vi "After Launch Init.vi"(8 "error in (no error)":errorcluster, 11 "CS++BaseActor in":refnum<class "CS++BaseActor.lvclass">) -> (0 "error out":errorcluster, 3 "CS++BaseActor out":refnum<class "CS++BaseActor.lvclass">)   [LabVIEW 2015, in "CS++BaseActor.lvlib" / "CS++BaseActor.lvclass"]
doc: "Use <b>After Launch init.vi</b> method only for sanity checks that are supposed to prevent the actor from launching if they fail. Use <B>this</B> method instead to initialize unique resources that must be released during the <b>Stop Core.vi</b> method. A corresponding high priority message will become dispatched before the <B>Actor Framework.lvlib:Actor.lvclass.Actor Core.vi</b> is called.\n\n<b>Derived classed should call the parent methode first</b> and their own initialization code after.\n\nRefer also to the ongoing discussion at https://decibel.ni.com/content/message/57394#57394."
uses:
  CS++BaseActor.lvclass
  <vilib>/ActorFramework/Actor/Actor.lvclass/Actor.ctl
  <vilib>/ActorFramework/Message Enqueuer/Message Enqueuer.lvclass/Message Enqueuer.ctl
  CS++BaseActor.lvclass/CS++BaseActor.ctl
  Libraries/Base/FGV Action.ctl
  CS++BaseActor Messages/Polling Start Stop Msg/Polling Start Stop Msg.lvclass/Polling Start Stop Msg.ctl
  CS++BaseActor Messages/Launch Associated GUI Msg/Launch Associated GUI Msg.lvclass/Launch Associated GUI Msg.ctl
  <vilib>/ActorFramework/Message Enqueuer/Init from Existing Queue.vi
  <vilib>/ActorFramework/Message Enqueuer/Enqueue.vi
  <vilib>/ActorFramework/Message Priority Queue/Priority Enqueue.vi
  CS++BaseActor Messages/Launch Associated GUI Msg/Launch Associated GUI Msg.lvclass
  <vilib>/ActorFramework/Message Enqueuer/Message Enqueuer.lvclass
  CS++BaseActor Messages/Polling Start Stop Msg/Polling Start Stop Msg.lvclass
  <vilib>/ActorFramework/Actor/Actor.lvclass
  Libraries/Base/CS++Base.lvlib
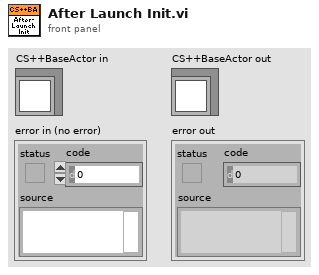
[diagram p1: front panel]
types:
  T1 = typedef "CS++Base.lvlib/FGV Action.ctl" = enum16{"add", "replace", "read", "remove", "reset", "get attributes"}
  T2 = cluster{"class name":string, "Self Enqueuer":refnum<class "Message Enqueuer.lvclass">}
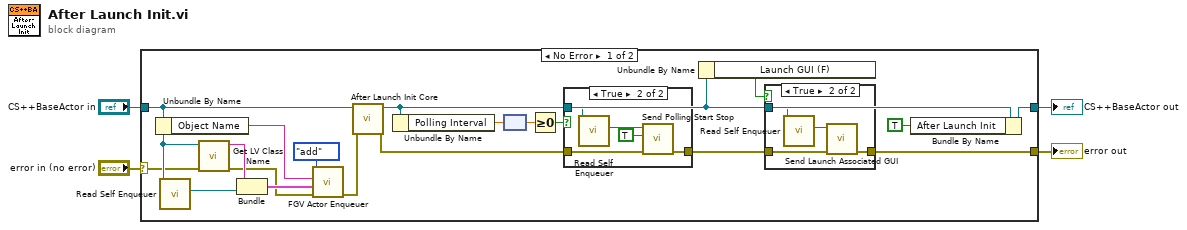
[diagram p0: block diagram]
diagram:
  n1 = case shown="No Error" "error in (no error)" {
    selector: "error in (no error)" -> [w14 w36]
    tunnel: [w7 w36] -> w3
    tunnel: [w23 w35] -> w1
    tunnel: "CS++BaseActor in" -> [w16 w35]
    frame No Error {
      n2 = Unbundle By Name(w16) -> ("Object Name"=w21:string)
      n3 = call <vilib>:"Read Self Enqueuer.vi"("Actor"=w16) -> ("Self Enqueuer"=w18:refnum<class "Message Enqueuer.lvclass">)  [unwired: 10 in]
      n4 = call <vilib>:"Get LV Class Name.vi"("error in (no error)"=w14, "object"=w16) -> ("error out"=w13:errorcluster, "class name"=w15:string)  [unwired: 8 in]
      n5 = Bundle("class name"=w15, "Self Enqueuer"=w18) -> (w17:T2)  [unwired: 1 in]
      n6 = call "FGV Actor Enqueuer.vi"("Error In"=w13, "Class & Enqueuer"=w17, "Actor Name"=w21, "Action (read)"=FGV_Action."add") -> ("Error Out"=w19:errorcluster)  [unwired: 3 in, 4 out]
      n7 = call-dynamic "After Launch Init Core.vi"("error in (no error)"=w19, "CS++BaseActor in"=w16) -> ("error out"=w12:errorcluster, "CS++BaseActor out"=w6:refnum<class "CS++BaseActor.lvclass">)  [unwired: 8 in]
      n8 = Unbundle By Name(w6) -> ("Polling Interval"=w10:dbl[unit])
      n9 = node(w10) -> (w9:dbl)
      n10 = Greater Or Equal To 0?(x=w9) -> (x >= 0?=w11:bool)
      n11 = case shown="True" w11 {
        tunnel: w6 -> [_ w29]
        tunnel: w12 -> [w24 w27]
        tunnel: [w24 w26] -> w8
        frame False {
        }
        frame True {
          n12 = call <vilib>:"Read Self Enqueuer.vi"("Actor"=w29) -> ("Self Enqueuer"=w28:refnum<class "Message Enqueuer.lvclass">)  [unwired: 10 in]
          n13 = call "Send Polling Start Stop.vi"("error in (no error)"=w27, "Start Polling"=TRUE, "Message Enqueuer"=w28) -> ("error out"=w26:errorcluster)  [unwired: 7 in, 1 out]
        }
      }
      n14 = Unbundle By Name(w6) -> ("Launch GUI (F)"=w5:bool)
      n15 = case shown="True" w5 {
        tunnel: w8 -> [w30 w33]
        tunnel: [w30 w32] -> w7
        tunnel: w6 -> [_ w31]
        frame False {
        }
        frame True {
          n16 = call <vilib>:"Read Self Enqueuer.vi"("Actor"=w31) -> ("Self Enqueuer"=w34:refnum<class "Message Enqueuer.lvclass">)  [unwired: 10 in]
          n17 = call "Send Launch Associated GUI.vi"("error in (no error)"=w33, "Message Enqueuer"=w34) -> ("error out"=w32:errorcluster)  [unwired: 8 in, 1 out]
        }
      }
      n18 = Bundle By Name(cluster=w6, "After Launch Init"=TRUE) -> (w23:refnum<class "CS++BaseActor.lvclass">)
    }
    frame Error {
    }
  }
  "error out" <- w3
  "CS++BaseActor out" <- w1
